vi "SimpleTempTest.vi"() -> ()   [LabVIEW 2019]
uses:
  <userlib>/MicroPython/VIs/uPythonX/uPythonX.xctl
panel:
  in  "Periperal demo":T1(xcontrol)={"Port"="Dylan pybd - ASRL117::INSTR", "All Code"="'''\nTaken from https://github.com/micropython/micropython/tree/master/examples/bluetooth\n\nimport ble_temperature as periph\nperiph.demo()\n'''\nfrom micropython import const\nimport struct, random, time\nimport bluetooth\n\nfrom temp2BLE import *\n\ndef Periph():\n    ble = bluetooth.BLE()\n    temp = Temp_Periph(ble)\n\n    t = 25\n    i = 0\n\n    while True:\n        # Write every second, notify every 10 seconds.\n        i = (i + 1) % 10\n        temp.set_temperature(t, notify=i == 0)\n        # Random walk the temperature.\n        t += random.uniform(-0.5, 0.5)\n        time.sleep_ms(1000)\n\nPeriph()"}
  in  "Central demo":T1(xcontrol)={"Port"="pyboard - ASRL96::INSTR", "All Code"="'''\nTaken from https://github.com/micropython/micropython/tree/master/examples/bluetooth\nimport ble_temperature_central as central\nimport bluetooth\ncentral.demo()\n\n'''\nfrom micropython import const\nimport struct, time\nimport bluetooth\n\nfrom temp2BLE import *\n\ndef Central():\n     ble = bluetooth.BLE()\n     central = Temp_Central(ble)\n\n     not_found = False\n\n     def on_scan(addr_type, addr, name):\n          if addr_type is not None:\n               print('Found sensor:', addr_type, addr, name)\n               central.connect()\n          else:\n               nonlocal not_found\n               not_found = True\n               print('No sensor found.')\n\n     central.scan(callback=on_scan)\n\n     # Wait for connection...\n     while not central.is_connected():\n          time.sleep_ms(100)\n          if not_found:\n               return\n\n     print('Connected')\n     \n     ''' print every 2 sec reading whatever is in the buffer\n     while central.is_connected():\n          central.read(callback=print)        # Explicitly issue reads, using \"print\" as the callback.\n          time.sleep_ms(2000)\n          '''\n     ''' Alternative to the above, just show the most recently notified value.\n     while central.is_connected():\n          print(central.value())\n          time.sleep_ms(2000)\n          '''\n     ''' or wait until notification\n     while central.is_connected():\n          central.on_notify(callback = print)\n     '''\n     while central.is_connected():\n\n\n     print('Disconnected')\n\nCentral()"}
  in  "tempBLE":T1(xcontrol)={"Port"="Dylan pybd - ASRL117::INSTR", "All Code"="'''\nTaken from https://github.com/micropython/micropython/tree/master/examples/bluetooth\n'''\nfrom micropython import const\nimport struct\nimport bluetooth\n\n# Advertising payloads are repeated packets of the following form:\n#   1 byte data length (N + 1)\n#   1 byte type (see constants below)\n#   N bytes type-specific data\n\n_ADV_TYPE_FLAGS = const(0x01)\n_ADV_TYPE_NAME = const(0x09)\n_ADV_TYPE_UUID16_COMPLETE = const(0x3)\n_ADV_TYPE_UUID32_COMPLETE = const(0x5)\n_ADV_TYPE_UUID128_COMPLETE = const(0x7)\n_ADV_TYPE_UUID16_MORE = const(0x2)\n_ADV_TYPE_UUID32_MORE = const(0x4)\n_ADV_TYPE_UUID128_MORE = const(0x6)\n_ADV_TYPE_APPEARANCE = const(0x19)\n\n_IRQ_CENTRAL_CONNECT                    = const(1 << 0)\n_IRQ_CENTRAL_DISCONNECT              = const(1 << 1)\n_IRQ_GATTS_WRITE                               = const(1 << 2)\n_IRQ_GATTS_READ_REQUEST              = const(1 << 3)\n_IRQ_SCAN_RESULT                              = const(1 << 4)\n_IRQ_SCAN_COMPLETE                        = const(1 << 5)\n_IRQ_PERIPHERAL_CONNECT              = const(1 << 6)\n_IRQ_PERIPHERAL_DISCONNECT        = const(1 << 7)\n_IRQ_GATTC_SERVICE_RESULT           = const(1 << 8)\n_IRQ_GATTC_CHARACTERISTIC_RESULT     = const(1 << 9)\n_IRQ_GATTC_DESCRIPTOR_RESULT     = const(1 << 10)\n_IRQ_GATTC_READ_RESULT                 = const(1 << 11)\n_IRQ_GATTC_WRITE_STATUS              = const(1 << 12)\n_IRQ_GATTC_NOTIFY                           = const(1 << 13)\n_IRQ_GATTC_INDICATE                        = const(1 << 14)\n_IRQ_ALL                                              = const(0xffff)\n\n\n# ---------- UUID Definitions Stuff ---------------\n\nENV_SENSE_UUID = bluetooth.UUID(0x181A)\nTEMP_UUID = bluetooth.UUID(0x2A6E)\n\nTEMP_CHAR = (TEMP_UUID, bluetooth.FLAG_READ|bluetooth.FLAG_NOTIFY,)\nENV_SENSE_SERVICE = (ENV_SENSE_UUID, (TEMP_CHAR,),)\n\nDESIRED_SERVICE_UUID =  ENV_SENSE_SERVICE \nDESIRED_CHAR_UUID = TEMP_UUID    # org.bluetooth.characteristic.temperature\n\n# org.bluetooth.characteristic.gap.appearance.xml\nADV_APPEARANCE_GENERIC_THERMOMETER = const(768)\nAPPEARANCE = ADV_APPEARANCE_GENERIC_THERMOMETER\n\n\n# ---------- Peripheral Stuff ---------------\n\nclass Temp_Periph:\n    def __init__(self, ble, name='mpy-temp'):\n        self._ble = ble\n        self._ble.active(True)\n        self._ble.irq(handler=self._irq)\n        ((self._handle,),) = self._ble.gatts_register_services((DESIRED_SERVICE_UUID,))\n        self._connections = set()\n        self._payload = advertising_payload(name=name, services=[ENV_SENSE_UUID], appearance=APPEARANCE)\n        self._advertise()\n\n    def _irq(self, event, data):\n        # Track connections so we can send notifications.\n        if event == _IRQ_CENTRAL_CONNECT:\n            conn_handle, _, _, = data\n            self._connections.add(conn_handle)\n        elif event == _IRQ_CENTRAL_DISCONNECT:\n            conn_handle, _, _, = data\n            self._connections.remove(conn_handle)\n            # Start advertising again to allow a new connection.\n            self._advertise()\n\n    def set_temperature(self, temp_deg_c, notify=False):\n        # Data is sint16 in degrees Celsius with a resolution of 0.01 degrees Celsius.\n        # Write the local value, ready for a central to read.\n        self._ble.gatts_write(self._handle, struct.pack('<h', int(temp_deg_c * 100)))\n        if notify:\n            for conn_handle in self._connections:\n                # Notify connected centrals to issue a read.\n                self._ble.gatts_notify(conn_handle, self._handle)\n\n    def _advertise(self, interval_us=500000):\n        self._ble.gap_advertise(interval_us, adv_data=self._payload)\n\n\n\n# ---------- Central Stuff ---------------\n\nclass Temp_Central:\n    def __init__(self, ble):\n        self._ble = ble\n        self._ble.active(True)\n        self._ble.irq(handler=self._irq)\n\n        self._reset()\n\n    def _reset(self):\n        # Cached name and address from a successful scan.\n        self._name = None\n        self._addr_type = None\n        self._addr = None\n\n        # Cached value (if we have one)\n        self._value = None\n\n        # Callbacks for completion of various operations.\n        # These reset back to None after being invoked.\n        self._scan_callback = None\n        self._conn_callback = None\n        self._read_callback = None\n\n        # Persistent callback for when new data is notified from the device.\n        self._notify_callback = None\n\n        # Connected device.\n        self._conn_handle = None\n        self._value_handle = None\n\n    def _irq(self, event, data):\n        if event == _IRQ_SCAN_RESULT:\n            addr_type, addr, connectable, rssi, adv_data = data\n            if connectable and ENV_SENSE_UUID in decode_services(adv_data):\n                # Found a potential device, remember it and stop scanning.\n                self._addr_type = addr_type\n                self._addr = bytes(addr) # Note: The addr buffer is owned by modbluetooth, need to copy it.\n                self._name = decode_name(adv_data) or '?'\n                self._ble.gap_scan(None)\n\n        elif event == _IRQ_SCAN_COMPLETE:\n            if self._scan_callback:\n                if self._addr:\n                    # Found a device during the scan (and the scan was explicitly stopped).\n                    self._scan_callback(self._addr_type, self._addr, self._name)\n                    self._scan_callback = None\n                else:\n                    # Scan timed out.\n                    self._scan_callback(None, None, None)\n\n        elif event == _IRQ_PERIPHERAL_CONNECT:\n            # Connect successful.\n            conn_handle, addr_type, addr, = data\n            if addr_type == self._addr_type and addr == self._addr:\n                self._conn_handle = conn_handle\n                self._ble.gattc_discover_services(self._conn_handle)\n\n        elif event == _IRQ_PERIPHERAL_DISCONNECT:\n            # Disconnect (either initiated by us or the remote end).\n            conn_handle, _, _, = data\n            if conn_handle == self._conn_handle:\n                # If it was initiated by us, it'll already be reset.\n                self._reset()\n\n        elif event == _IRQ_GATTC_SERVICE_RESULT:\n            # Connected device returned a service.\n            conn_handle, start_handle, end_handle, uuid = data\n            if conn_handle == self._conn_handle and uuid == ENV_SENSE_UUID:\n                self._ble.gattc_discover_characteristics(self._conn_handle, start_handle, end_handle)\n\n        elif event == _IRQ_GATTC_CHARACTERISTIC_RESULT:\n            # Connected device returned a characteristic.\n            conn_handle, def_handle, value_handle, properties, uuid = data\n            if conn_handle == self._conn_handle and uuid == TEMP_UUID:\n                self._value_handle = value_handle\n                # We've finished connecting and discovering device, fire the connect callback.\n                if self._conn_callback:\n                    self._conn_callback()\n\n        elif event == _IRQ_GATTC_READ_RESULT:\n            # A read completed successfully.\n            conn_handle, value_handle, char_data = data\n            if conn_handle == self._conn_handle and value_handle == self._value_handle:\n                self._update_value(char_data)\n                if self._read_callback:\n                    self._read_callback(self._value)\n                    self._read_callback = None\n\n        elif event == _IRQ_GATTC_NOTIFY:\n            # The ble_temperature.py demo periodically notifies its value.\n            conn_handle, value_handle, notify_data = data\n            if conn_handle == self._conn_handle and value_handle == self._value_handle:\n                self._update_value(notify_data)\n                if self._notify_callback:\n                    self._notify_callback(self._value)\n\n\n    # Returns true if we've successfully connected and discovered characteristics.\n    def is_connected(self):\n        return self._conn_handle is not None and self._value_handle is not None\n\n    # Find a device advertising the environmental sensor service.\n    def scan(self, callback=None):\n        self._addr_type = None\n        self._addr = None\n        self._scan_callback = callback\n        self._ble.gap_scan(2000, 20000, 30000) # for 2 sec, scan every 30 msec for 20 msec\n\n    # Connect to the specified device (otherwise use cached address from a scan).\n    def connect(self, addr_type=None, addr=None, callback=None):\n        self._addr_type = addr_type or self._addr_type\n        self._addr = addr or self._addr\n        self._conn_callback = callback\n        if self._addr_type is None or self._addr is None:\n            return False\n        self._ble.gap_connect(self._addr_type, self._addr)\n        return True\n\n    # Disconnect from current device.\n    def disconnect(self):\n        if not self._conn_handle:\n            return\n        self._ble.gap_disconnect(self._conn_handle)\n        self._reset()\n\n    # Issues an (asynchronous) read, will invoke callback with data.\n    def read(self, callback):\n        if not self.is_connected():\n            return\n        self._read_callback = callback\n        self._ble.gattc_read(self._conn_handle, self._value_handle)\n\n    # Sets a callback to be invoked when the device notifies us.\n    def on_notify(self, callback):\n        self._notify_callback = callback\n\n    def _update_value(self, data):\n        # Data is sint16 in degrees Celsius with a resolution of 0.01 degrees Celsius.\n        self._value = struct.unpack('<h', data)[0] / 100\n        return self._value\n\n    def value(self):\n        return self._value\n\n# ---------- ADVERTISING Stuff ---------------\n\n\n# Generate a payload to be passed to gap_advertise(adv_data=...).\ndef advertising_payload(limited_disc=False, br_edr=False, name=None, services=None, appearance=0):\n    payload = bytearray()\n\n    def _append(adv_type, value):\n        nonlocal payload\n        payload += struct.pack('BB', len(value) + 1, adv_type) + value\n\n    _append(_ADV_TYPE_FLAGS, struct.pack('B', (0x01 if limited_disc else 0x02) + (0x00 if br_edr else 0x04)))\n\n    if name:\n        _append(_ADV_TYPE_NAME, name)\n\n    if services:\n        for uuid in services:\n            b = bytes(uuid)\n            if len(b) == 2:\n                _append(_ADV_TYPE_UUID16_COMPLETE, b)\n            elif len(b) == 4:\n                _append(_ADV_TYPE_UUID32_COMPLETE, b)\n            elif len(b) == 16:\n                _append(_ADV_TYPE_UUID128_COMPLETE, b)\n\n    # See org.bluetooth.characteristic.gap.appearance.xml\n    _append(_ADV_TYPE_APPEARANCE, struct.pack('<h', appearance))\n\n    return payload\n\n\ndef decode_field(payload, adv_type):\n    i = 0\n    result = []\n    while i + 1 < len(payload):\n        if payload[i + 1] == adv_type:\n            result.append(payload[i + 2:i + payload[i] + 1])\n        i += 1 + payload[i]\n    return result\n\n\ndef decode_name(payload):\n    n = decode_field(payload, _ADV_TYPE_NAME)\n    return str(n[0], 'utf-8') if n else ''\n\n\ndef decode_services(payload):\n    services = []\n    for u in decode_field(payload, _ADV_TYPE_UUID16_COMPLETE):\n        services.append(bluetooth.UUID(struct.unpack('<h', u)[0]))\n    for u in decode_field(payload, _ADV_TYPE_UUID32_COMPLETE):\n        services.append(bluetooth.UUID(struct.unpack('<d', u)[0]))\n    for u in decode_field(payload, _ADV_TYPE_UUID128_COMPLETE):\n        services.append(bluetooth.UUID(u))\n    return services\n\n\ndef payloadDemo():\n    payload = advertising_payload(name='micropython', services=[bluetooth.UUID(0x181A), bluetooth.UUID('6E400001-B5A3-F393-E0A9-E50E24DCCA9E')])\n    print(payload)\n    print(decode_name(payload))\n    print(decode_services(payload))\n\n"}
  in  "PyBoard 2":T1(xcontrol)={"Port"="Dylan pybd - ASRL117::INSTR", "All Code"="'''\nmac address b'HJ0\\x01pB'\n'''\n\nimport bluetooth,utime\n\nble = bluetooth.BLE()\nble.active(True)\n\nble.config('mac')\n\ndef bt_callback(event, data):\n    print('bt_irq: ', event, data)\n        \nble.irq(bt_callback)"}
  in  "PyBoard 1":T1(xcontrol)={"Port"="pyboard - ASRL96::INSTR", "All Code"="'''\nmac address of pybd: b'HJ0\\x01o\\xf2' or 48:4A:01:6F:F2\n     '''\n     '''\nHR_UUID = ubluetooth.UUID(0x180D)\nHR_CHAR = (ubluetooth.UUID(0x2A37), ubluetooth.FLAG_READ | ubluetooth.FLAG_NOTIFY,)\nHR_SERVICE = (HR_UUID, (HR_CHAR,),)\nSERVICES = (HR_SERVICE, )\n(hr,) = bt.gatts_register_services(SERVICES)\n'''\n\nimport bluetooth,utime\n\nble = bluetooth.BLE()\nble.active(True)\n\nLWP_CHAR = (\n    bluetooth.UUID('00001624-1212-EFDE-1623-785FEABCD123'),\n    bluetooth.FLAG_WRITE | bluetooth.FLAG_NOTIFY,\n    # List of descriptors\n    (   \n        # CCCD\n        (bluetooth.UUID(0x2902), bluetooth.FLAG_READ | bluetooth.FLAG_WRITE), \n    )\n)   \nLPF2_SERVICE = (bluetooth.UUID('00001623-1212-EFDE-1623-785FEABCD123'), (LWP_CHAR,))\nALL_SERVICES = (LPF2_SERVICE,)\n\n(lwp_char, lwp_descr), = ble.gatts_register_services(ALL_SERVICES)\n\ndef bt_irq(x, y):\n    print('bt_irq', x, y)\n        \nble.irq(bt_irq)\n\ndef adv_encode_name(name):\n    name = bytes(name, 'ascii')\n    return bytearray((len(name) + 1, 0x09)) + name\n\ndef adv(name):\n    ble.gap_advertise(100_000, adv_data=b'\\x02\\x01\\x06' + adv_encode_name(name))\n\nadv('pybd-lpf2')\n\nutime.sleep(5)   # wait for pyboard to get ready and connect\n\nble.gatts_notify(64, lwp_char, 'from pybd')\n\nble.gatts_read(lwp_char)"}
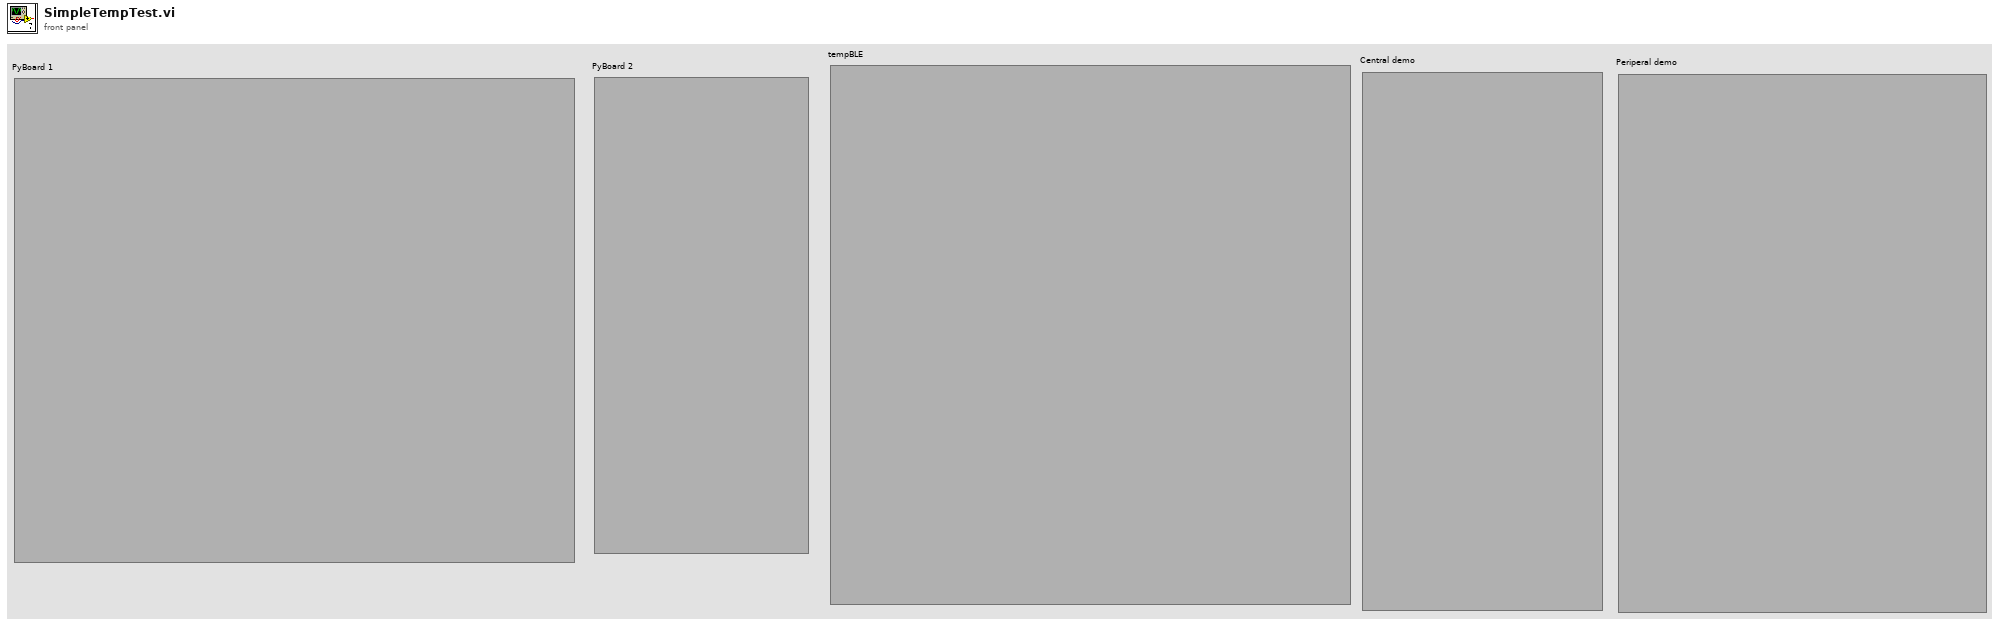
[diagram p1: front panel]
types:
  T1 = cluster{"Port":refnum<visa-resource-name>, "All Code":string}
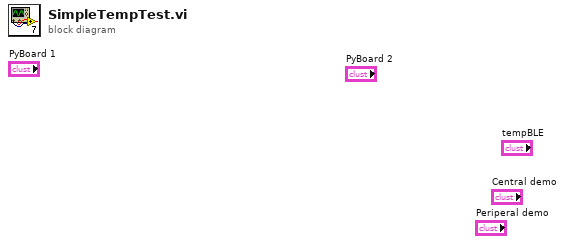
[diagram p0: block diagram]
diagram:
